vi "Evaluate Directional Derivative.vi"(1 "Direction v=(v_1, ..., v_n)":dbl[](array[numeric]), 2 "Point x=(x_1, ..., x_n)":dbl[](array[numeric]), 4 "Function Reference":refnum<vi>) -> (0 "Grad_v f(x)":dbl format="%.2f")   [LabVIEW 2020, in "Automatic Differentiation.lvlib"]
uses:
  Automatic Differentiation.lvlib
  classes/Dual/Dual.lvclass
  <vilib>/Analysis/_algsub.llb/Vector Norm Type.ctl
  classes/Dual/Dual.lvclass/Dual.ctl
  <vilib>/Analysis/baseanly.llb/Real Dot Product.vi
  <vilib>/Analysis/_algsub.llb/Real Vector Norm.vi
  Evaluate Gradient.vi/3428a883-4abf-4854-9978-3fd53a24097c.vi
  classes/Dual/Add infinitesimal to Double.vi
  classes/Dual/Read Dual Part.vi
  Evaluate Gradient.vi/3428a883-4abf-4854-9978-3fd53a24097c.vi/5957e011-cf56-4527-b6ed-13c3a4ca997b.vi
  classes/Dual/Write a.vi
  <vilib>/Analysis/NI_AALBase.lvlib
  <vilib>/Analysis/NI_AALPro.lvlib
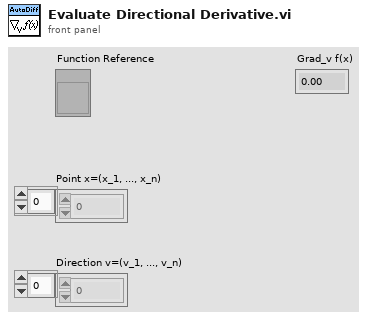
[diagram p1: front panel]
types:
  T1 = typedef "NI_AALPro.lvlib/Vector Norm Type.ctl" = u16
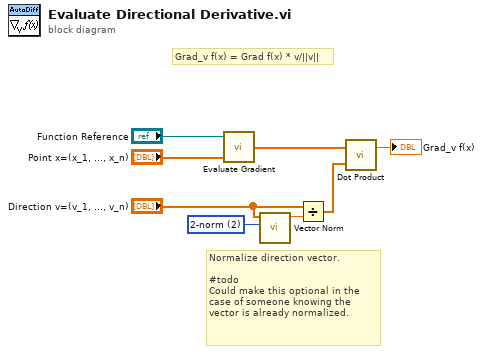
[diagram p0: block diagram]
diagram:
  w7 = T1 2 items=["1-norm"=1, "2-norm"=2, "Inf-norm"=3, "-Inf-norm"=4, "User Defined"=5] ("norm type")
  # "Grad_v f(x) = Grad f(x) * v/||v||"
  # "Normalize direction vector.\n\n#todo\nCould make this optional in the case of someone knowing the vector is already normalized."
  n1 = call "Evaluate Gradient.vi"("Point (x_1, ..., x_n)"="Point x=(x_1, ..., x_n)", "Function Reference"="Function Reference") -> ("Gradient"=w1:dbl[])  [unwired: 2 in]
  n2 = call-poly <vilib>:"Vector Norm.vi"("norm type"=w7, "Input Vector"="Direction v=(v_1, ..., v_n)") -> ("norm"=w6:dbl)  [unwired: 8 in, 1 out]
  n3 = Divide(x="Direction v=(v_1, ..., v_n)", y=w6) -> (x/y=w4:dbl[])
  n4 = call-poly <vilib>:"Dot Product.vi"("Y Vector"=w4, "X Vector"=w1) -> ("X * Y"=→"Grad_v f(x)":dbl)  [unwired: 1 out]
